vi "Report.vi"() -> ()   [LabVIEW 2023]
uses:
  <vilib>/addons/database/Auxilliary.llb/DB Tools Cursor Type.ctl
  <vilib>/addons/database/Connection.llb/DB Tools Open Connec (Path).vi
  <vilib>/addons/database/Connection.llb/Conn Execute.vi
  <vilib>/addons/database/Recordset.llb/Rec Fetch Recordset Data (R).vi
  <vilib>/addons/database/Recordset.llb/Rec Destroy - Connection.vi
  <vilib>/addons/database/_DB Variant To Data/Database Variant To Data.xnode
  <vilib>/addons/database/NI_Database_API.lvlib
panel:
  in  "Call_Close":bool
  out "Records":string[][](table)
  in  "Fetch":bool
  in  "stop":bool
  # "SERvice call CLOSE"
  # "UTKARSH ENTERPRISES"
  # "Developed By- Samarth Wagh (waghsamarth@gmail.com) 7972965098"
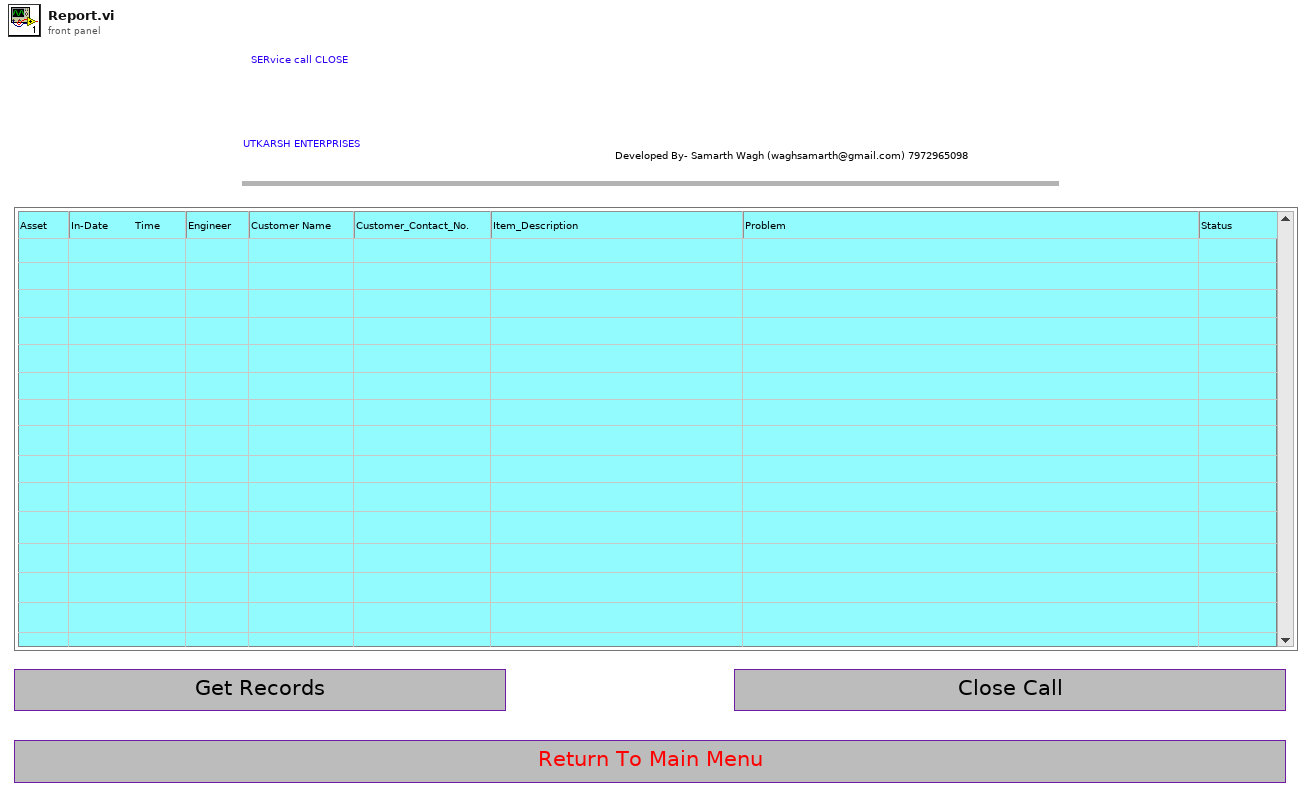
[diagram p1: front panel]
types:
  T1 = typedef "NI_Database_API.lvlib/DB Tools Cursor Type.ctl" = enum16{"forward-only", "keyset", "dynamic", "static"}
  T2 = typedef "LVRowAndColumnTypeDef.ctl" = cluster{"Row":i32, "Column":i32}
  T3 = typedef "NI_Database_API.lvlib/Conn ObjectReference.ctl" = refnum<k1>
  T4 = typedef "NI_Database_API.lvlib/Rec ObjectReference.ctl" = refnum<k1>
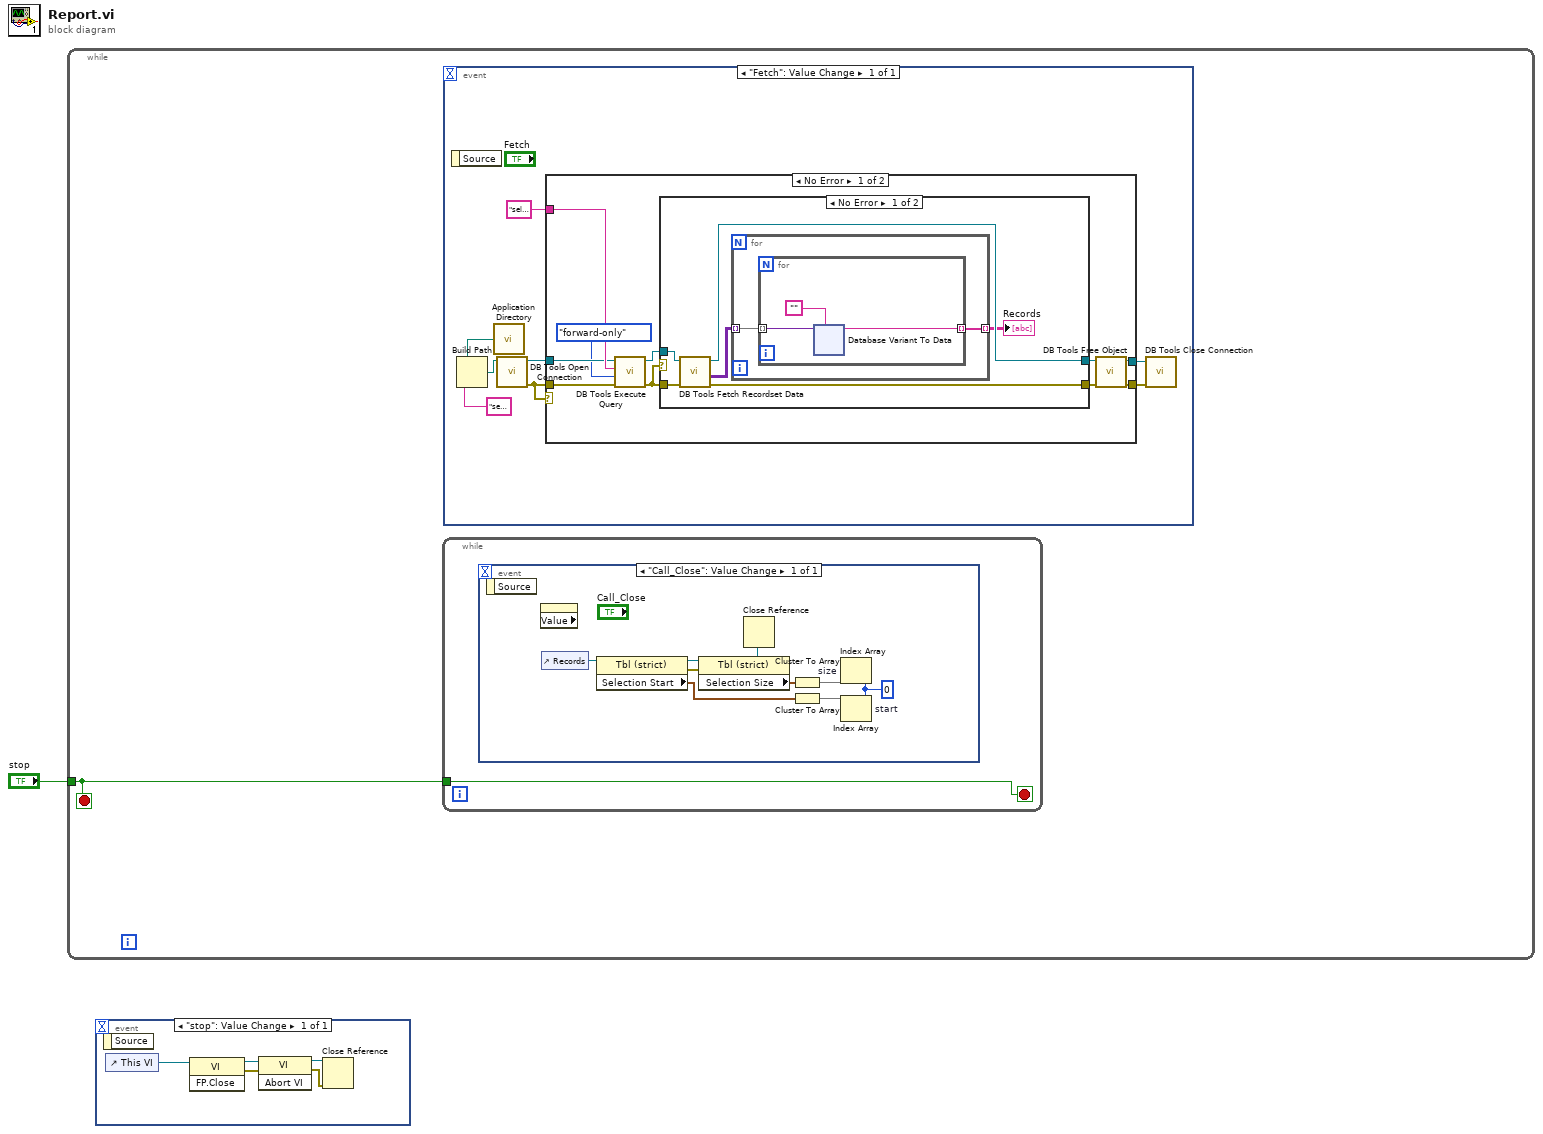
[diagram p0: block diagram]
diagram:
  n1 = while {
    tunnel: "stop" -> [w2]
    stop <- w2 stop-if-true
    n2 = while {
      tunnel: w2 -> [w3]
      stop <- w3 stop-if-true
      n3 = event shown="[0] \"Call_Close\": Value Change" {
        selector: _ -> [_]
        dyn-events: _ -> [_]
        timeout: _ -> [_]
        event "Call_Close": Value Change {
          w6 = 0 ("index")
          n4 = event-data() -> ()  [unwired: 1 in, 1 out]
          n5 = property on="Records" class="Tbl (strict)" props=["Value"]() -> ()  [unwired: 2 in, 3 out]
          n6 = control-ref of="Records"() -> (w12:refnum<vi>)
          n7 = property class="Tbl (strict)"(reference=w12) -> (reference out=w11:refnum<vi>, error out=w10:errorcluster, "Selection Start"=w4:T2)  [unwired: 1 in]
          n8 = property class="Tbl (strict)"(reference=w11, error in=w10) -> (reference out=w9:refnum<vi>, "Selection Size"=w5:T2)  [unwired: 1 out]
          n9 = Close Reference(reference=w9) -> ()  [unwired: 1 in, 1 out]
          n10 = Cluster To Array(cluster=w5) -> (array=w8:i32[])
          n11 = Cluster To Array(cluster=w4) -> (array=w7:i32[])
          n12 = Index Array "size"(array=w8, index=w6) -> ()  [unwired: 1 out]
          n13 = Index Array "start"(array=w7, index=w6) -> ()  [unwired: 1 out]
        }
      }
    }
    n14 = event shown="[0] \"Fetch\": Value Change" {
      selector: _ -> [_]
      dyn-events: _ -> [_]
      timeout: _ -> [_]
      event "Fetch": Value Change {
        n15 = event-data() -> ()  [unwired: 1 in, 1 out]
        n16 = call <vilib>:"Application Directory.vi"() -> ("Application Directory"=w17:path)
        n17 = Build Path(base path=w17, name or relative path="service_calls_entries.udl") -> (appended path=w15:path)
        n18 = call-poly <vilib>:"DB Tools Open Connection.vi"("connection information"=w15) -> ("error out"=w19:errorcluster, "connection reference"=w20:T3)  [unwired: 7 in]
        n19 = case shown="No Error" w19 {
          tunnel: "select * from Service_Calls_Entry" -> [w30 _]
          tunnel: [w25 w76] -> w13
          tunnel: [w23 w77] -> w18
          tunnel: w19 -> [w28 w76]
          tunnel: w20 -> [w27 w77]
          frame No Error {
            n20 = call-poly <vilib>:"DB Tools Execute Query.vi"("error in (no error)"=w28, "cursor type"=DB_Tools_Cursor_Type."forward-only", "SQL query"=w30, "connection reference"=w27) -> ("error out"=w26:errorcluster, "recordset reference"=w29:T4)  [unwired: 4 in]
            n21 = case shown="No Error" w26 {
              tunnel: [w33 w75] -> w24
              tunnel: [w34 w74] -> w22
              tunnel: w26 -> [w36 w75]
              tunnel: w29 -> [w35 w74]
              frame No Error {
                n22 = call-poly <vilib>:"DB Tools Fetch Recordset Data.vi"("error in (no error)"=w36, "recordset reference"=w35) -> ("error out"=w33:errorcluster, "recordset data"=w32:variant[][], "recordset reference out"=w34:T4)  [unwired: 3 in]
                n23 = for {
                  tunnel: w32 -> [w38] mode=indexing
                  tunnel: [w37] -> w31 mode=indexing
                  n24 = for {
                    tunnel: w38 -> [w41] mode=indexing
                    tunnel: [w39] -> w37 mode=indexing
                    n25 = xnode "Database Variant To Data"("database variant"=w41, "type"="") -> ("data"=w39:string)  [unwired: 1 in, 1 out]
                  }
                }
                "Records" <- w31
              }
              frame Error {
              }
            }
            n26 = call-poly <vilib>:"DB Tools Free Object.vi"("error in (no error)"=w24, "recordset reference"=w22) -> ("error out"=w25:errorcluster, "connection reference"=w23:T3)  [unwired: 8 in]
          }
          frame Error {
          }
        }
        n27 = call <vilib>:"DB Tools Close Connection.vi"("error in (no error)"=w13, "connection reference"=w18) -> ()  [unwired: 5 in, 1 out]
      }
    }
  }
  n28 = event shown="[0] \"stop\": Value Change" {
    selector: _ -> [_]
    dyn-events: _ -> [_]
    timeout: _ -> [_]
    event "stop": Value Change {
      n29 = event-data() -> ()  [unwired: 1 in, 1 out]
      n30 = control-ref of="This VI"() -> (w80:refnum<vi>)
      n31 = invoke class="VI" method="FP.Close"(reference=w80) -> (reference out=w79:refnum<vi>, error out=w78:errorcluster)  [unwired: 2 in, 1 out]
      n32 = invoke class="VI" method="Abort VI"(reference=w79, error in=w78) -> (reference out=w82:refnum<vi>, error out=w81:errorcluster)  [unwired: 1 in, 1 out]
      n33 = Close Reference(reference=w82, error in (no error)=w81) -> ()  [unwired: 1 out]
    }
  }
